vi "Config_CheckHardware.vi"(5 "Status Ref":refnum<vi>, 7 "HM 8119":refnum<vi>, 8 "error in (no error)":errorcluster, 10 "Config Cluster":T1={"General"={"Config.ini"=path "", "Default Logging Path"=path ""}, "Hardware"={"Measure Rate (1/s)"=0, "HP DMM VISA"="", "LS 335 VISA"="", "HP DM"={"Range"=enum."Autorange", "Autozero"=FALSE, "Display"=enum."3 1/2 Digit", "Blank LCD"=FALSE}}, "Operation"={"Operation Mode"=enum."Idle-Off", "Status"="", "NewLog?"=FALSE, "OvenWarn"=FALSE}}) -> (0 "error out":errorcluster, 1 "Connected?":bool, 2 "Config Cluster Out":T1={"General"={"Config.ini"=path "", "Default Logging Path"=path ""}, "Hardware"={"Measure Rate (1/s)"=0, "HP DMM VISA"="", "LS 335 VISA"="", "HP DM"={"Range"=enum."Autorange", "Autozero"=FALSE, "Display"=enum."3 1/2 Digit", "Blank LCD"=FALSE}}, "Operation"={"Operation Mode"=enum."Idle-Off", "Status"="", "NewLog?"=FALSE, "OvenWarn"=FALSE}})   [LabVIEW 2021]
uses:
  Config_Cluster.ctl
  Mode_Enum.ctl
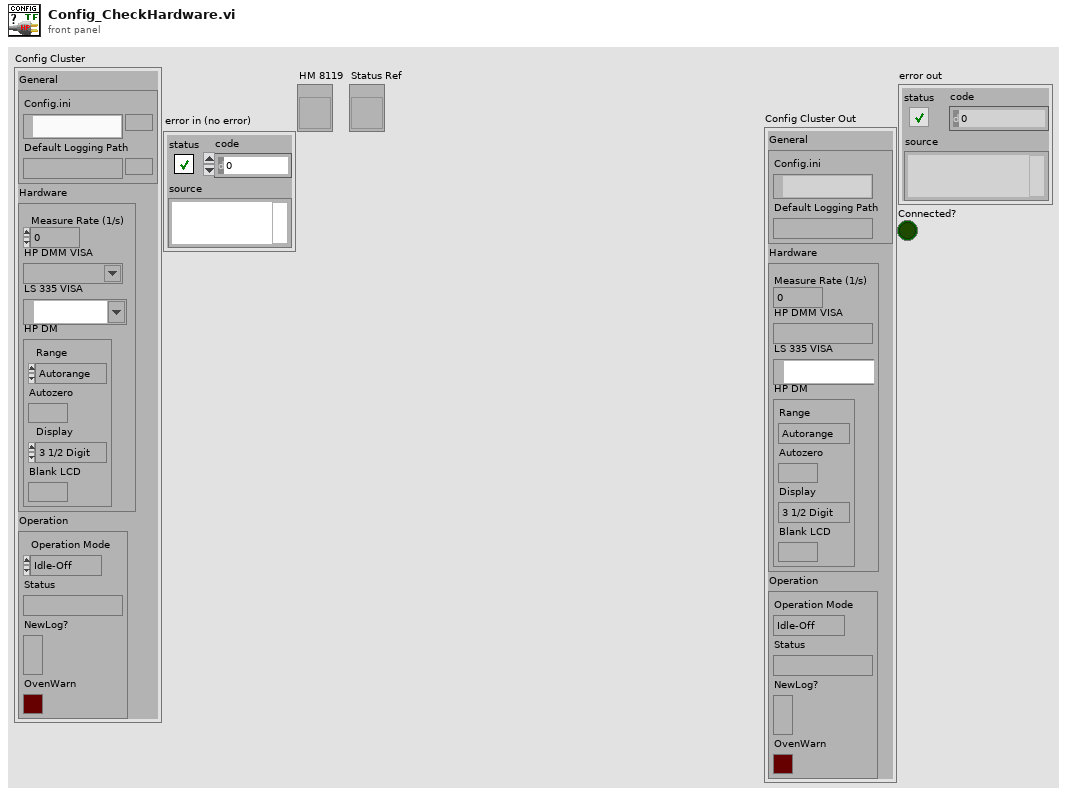
[diagram p1: front panel]
types:
  T1 = typedef "Config_Cluster.ctl" = cluster{"General":cluster{"Config.ini":path, "Default Logging Path":path}, "Hardware":cluster{"Measure Rate (1/s)":i32, "HP DMM VISA":refnum<visa-resource-name>, "LS 335 VISA":refnum<visa-resource-name>, "HP DM":cluster{"Range":enum16{"Autorange", "30mV", "300mV", "3V", "30V"}, "Autozero":bool, "Display":enum16{"3 1/2 Digit", "4 1/2 Digit", "5 1/2 Digit"}, "Blank LCD":bool}}, "Operation":cluster{"Operation Mode":T2, "Status":string, "NewLog?":bool, "OvenWarn":bool}}
  T2 = typedef "Mode_Enum.ctl" = enum16{"OvenNRDY", "Logging", "Idle-Off", "Idle"}
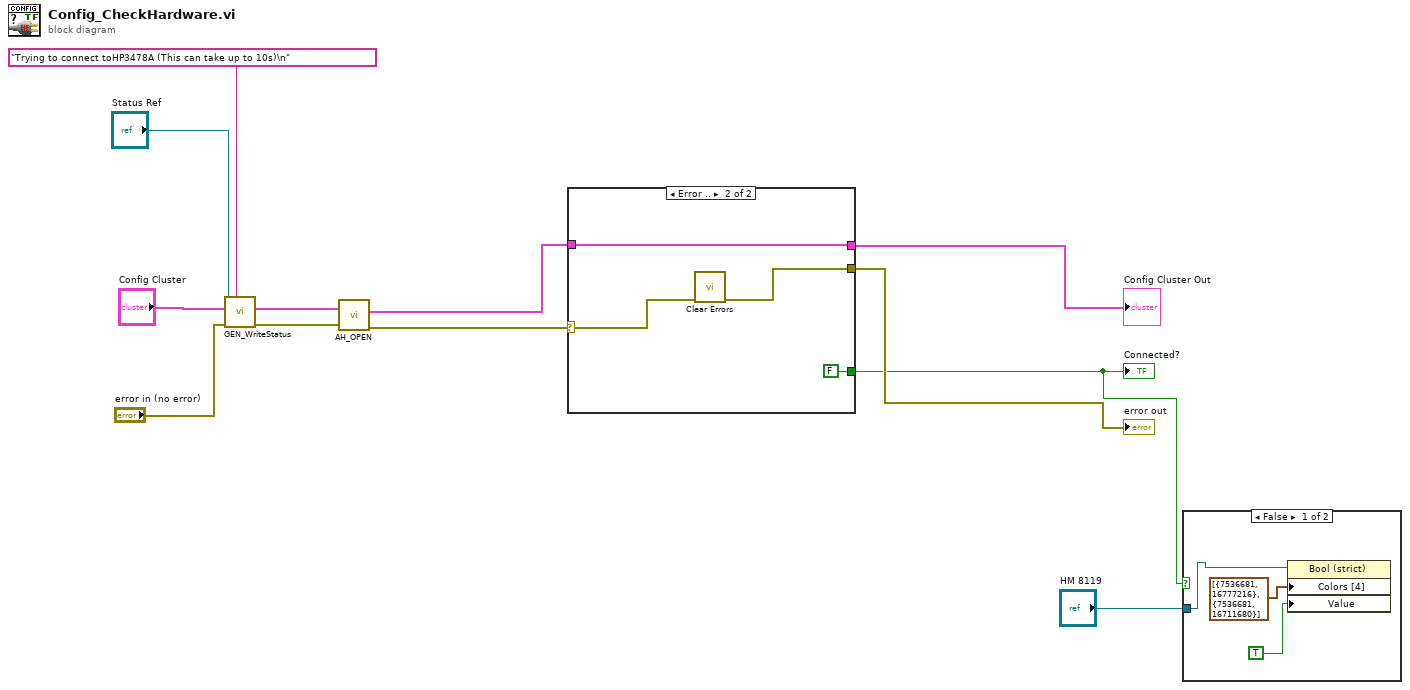
[diagram p0: block diagram]
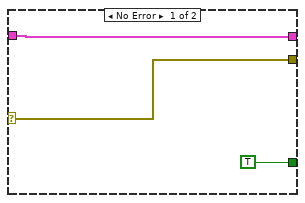
[diagram p2: hidden frame]
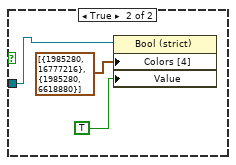
[diagram p3: hidden frame]
diagram:
  n1 = call "GEN_WriteStatus.vi"("Input String"="Trying to connect toHP3478A (This can take up to 10s)\n", "error in (no error)"="error in (no error)", "Config_Cluster"="Config Cluster", "Status Ref"="Status Ref") -> ("error out"=w4:errorcluster, "Config_Cluster Out"=w5:T1)  [unwired: 6 in]
  n2 = call "AH_OPEN.vi"("error in (no error)"=w4, "Configuration Cluster"=w5) -> ("error out"=w3:errorcluster, "Configuration Cluster Out"=w2:T1)  [unwired: 8 in]
  n3 = case shown="Error .." w3 {
    selector: w3 -> [w14 w19]
    tunnel: w2 -> [w15 w16]
    tunnel: [w15 w16] -> w1
    tunnel: [w14 w18] -> w12
    tunnel: [TRUE FALSE] -> w11
    frame No Error {
    }
    frame Error {
      n4 = call <vilib>:"Clear Errors.vi"("error in (no error)"=w19) -> ("error out"=w18:errorcluster)  [unwired: 5 in, 1 out]
    }
  }
  "Config Cluster Out" <- w1
  "error out" <- w12
  "Connected?" <- w11
  n5 = case shown="False" w11 {
    tunnel: "HM 8119" -> [w20 w23]
    frame False {
      n6 = property class="Bool (strict)"(reference=w20, "Colors [4]"=cluster{u32, u32}[] [{7536681, 16777216}, {7536681, 16711680}], "Value"=TRUE) -> ()  [unwired: 1 in, 2 out]
    }
    frame True {
      n7 = property class="Bool (strict)"(reference=w23, "Colors [4]"=cluster{u32, u32}[] [{1985280, 16777216}, {1985280, 6618880}], "Value"=TRUE) -> ()  [unwired: 1 in, 2 out]
    }
  }
